vi "Configuration Test.vi"() -> ()   [LabVIEW 2018, in "EMS Generic Actor.lvlib" / "EMS Generic.lvclass"]
uses:
  EMS Generic.lvclass
  EMS User Interface Actor/EMS User Interface/Controls/Configuration/Config PCC Controller.ctl
  EMS User Interface Actor/EMS User Interface/Controls/Configuration/Config VF Controller.ctl
  EMS User Interface Actor/EMS User Interface/EMS User Interface.lvclass
  <vilib>/Utility/config.llb/NI_LVConfig.lvlib
panel:
  out "Array":i32[](array[numeric])
  out "data 4":T1
  out "data 3":T2
  out "type string":i16[](array[numeric]) format="%04x"
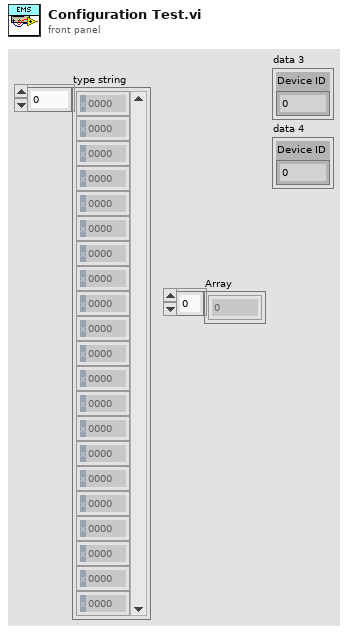
[diagram p1: front panel]
types:
  T1 = typedef "EMS User Interface Actor.lvlib/EMS User Interface.lvclass/Config VF Controller.ctl" = cluster{"Device ID":u64}
  T2 = typedef "EMS User Interface Actor.lvlib/EMS User Interface.lvclass/Config PCC Controller.ctl" = cluster{"Device ID":u64}
  T3 = cluster{u64, u16, dbl, dbl, dbl, dbl, dbl, dbl, dbl[], dbl[], dbl[], dbl[], dbl, dbl, dbl, dbl}[]
  T4 = typedef "NI_LVConfig.lvlib/Config Data RefNum.ctl" = refnum<k1>
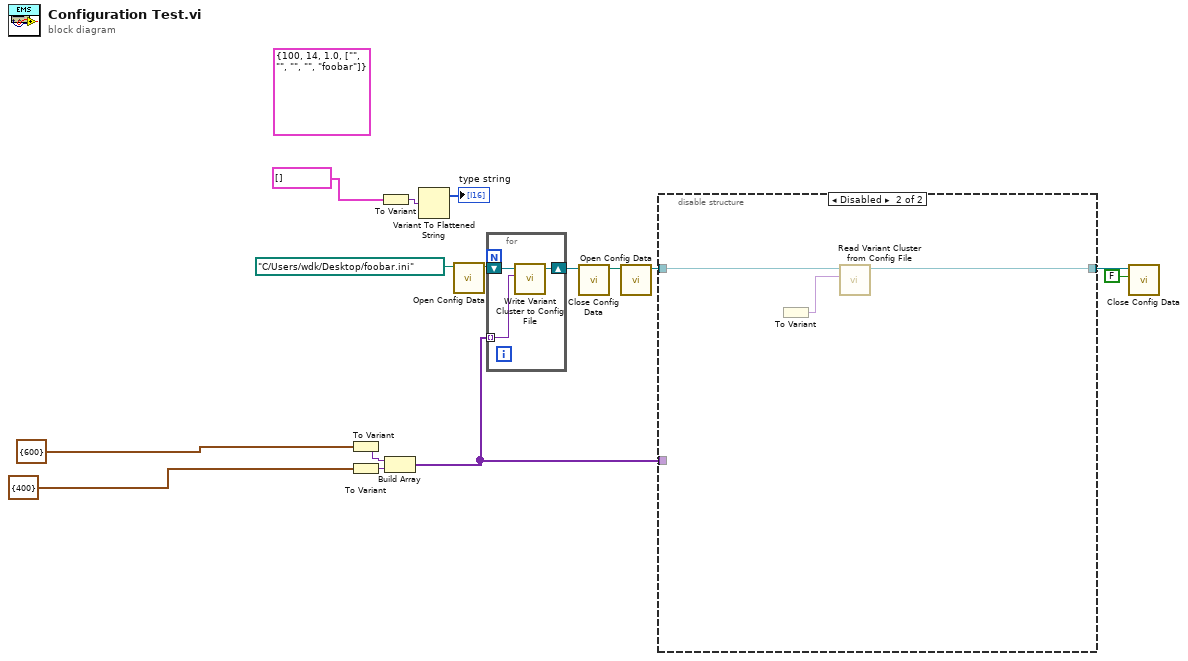
[diagram p0: block diagram]
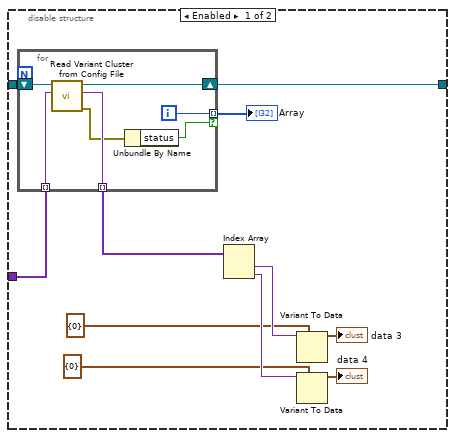
[diagram p2: hidden frame]
diagram:
  (unwired) cluster{u64, u16, dbl, string[]} {100, 14, 1.0, ["", "", "", "", "foobar"]}
  n1 = To Variant(anything=T2 {"Device ID"=600} ("PCC Controller")) -> (Variant=w11:variant)
  n2 = To Variant(anything=T1 {"Device ID"=400} ("V/F Controller")) -> (Variant=w14:variant)
  n3 = To Variant(anything=T3 []) -> (Variant=w7:variant)
  n4 = Build Array(w11, w14) -> (w5:variant[])
  n5 = Variant To Flattened String(Variant=w7) -> (1:→"type string":i16[])  [unwired: 1 out]
  n6 = call <vilib>:"Open Config Data.vi"("configuration file path"=path "C:/Users/wdk/Desktop/foobar.ini") -> ("refnum"=w15:T4)  [unwired: 8 in, 2 out]
  n7 = for {
    tunnel: w5 -> [w16] mode=indexing
    shift-right: [w17] -> w13
    shift-left: w15 -> [w18]
    n8 = call "Write Variant Cluster to Config File.vi"("Variant Configuration Object"=w16, "Config Refnum in"=w18) -> ("Config Refnum out"=w17:T4)  [unwired: 8 in, 1 out]
  }
  n9 = call <vilib>:"Close Config Data.vi"("refnum"=w13) -> ("file path"=w6:path)  [unwired: 9 in, 1 out]
  n10 = call <vilib>:"Open Config Data.vi"("configuration file path"=w6) -> ("refnum"=w3:T4)  [unwired: 8 in, 2 out]
  n11 = disable-structure shown="Disabled" {
    disable-tunnel: w5 -> [w29 _]
    disable-tunnel: w3 -> [w28 w40]
    disable-tunnel: [w19 w39] -> w1
    frame Enabled {
      n12 = for {
        tunnel: w29 -> [w34] mode=indexing
        shift-right: [w35] -> w19
        shift-left: w28 -> [w36]
        tunnel: [w33] -> w27 mode=indexing
        tunnel: [w32] -> w20 mode=indexing if=w30
        i -> [w32]
        n13 = call "Read Variant Cluster from Config File.vi"("Variant Cluster in"=w34, "Config Refnum in"=w36) -> ("error out"=w31:errorcluster, "Variant Cluster out"=w33:variant, "Config Refnum out"=w35:T4)  [unwired: 6 in, 1 out]
        n14 = Unbundle By Name(w31) -> ("status"=w30:bool)
      }
      "Array" <- w20
      n15 = Index Array(array=w27) -> (element #1=w26:variant, element #2=w25:variant)  [unwired: 2 in]
      n16 = Variant To Data(type=T2 {"Device ID"=0} ("PCC Controller"), Variant=w26) -> (data=→"data 3":T2)  [unwired: 1 in, 1 out]
      n17 = Variant To Data(type=T1 {"Device ID"=0} ("V/F Controller"), Variant=w25) -> (data=→"data 4":T1)  [unwired: 1 in, 1 out]
    }
    frame Disabled {
      n18 = To Variant() -> (anything=w37:cluster{}, Variant=w38:variant)
      n19 = call "Read Variant Cluster from Config File.vi"("Variant Cluster in"=w38, "Config Refnum in"=w40) -> ("Config Refnum out"=w39:T4)  [unwired: 6 in, 3 out]
    }
  }
  n20 = call <vilib>:"Close Config Data.vi"("write file if changed (T)"=FALSE, "refnum"=w1) -> ()  [unwired: 8 in, 2 out]
